vi "SET_FIRE_CUSTOM.vi"(10 "argv":string[](array[string]), 11 "args":u8) -> ()   [LabVIEW 2011]
uses:
  <vilib>/Rock Robotics/WPI/DriverStation/WPI_DriverStationStatusErrorCache.ctl
  Auto_Conf.vi
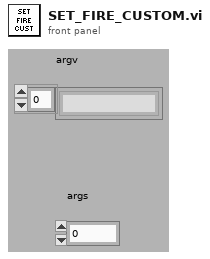
[diagram p1: front panel]
types:
  T1 = typedef "WPI_DriverStationStatusErrorCache.ctl" = enum16{"Get", "Set"}
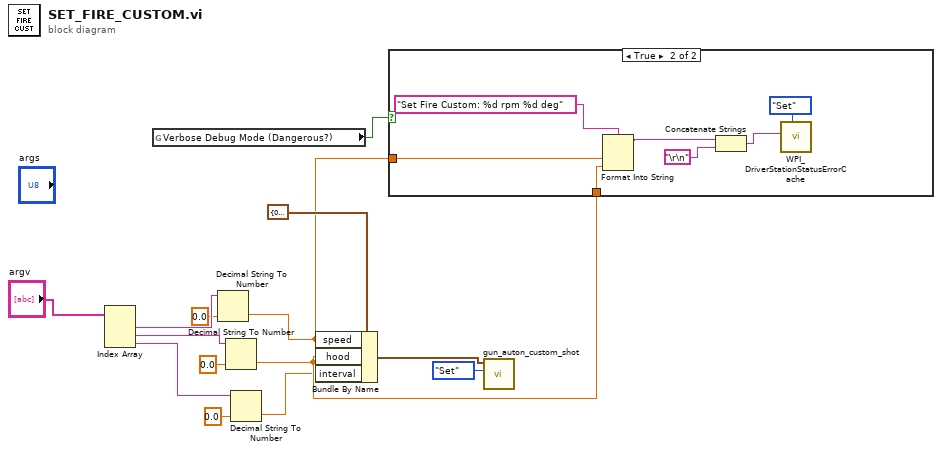
[diagram p0: block diagram]
diagram:
  n1 = Index Array(array="argv") -> (element #1=w13:string, element #2=w10:string, element #3=w2:string)  [unwired: 3 in]
  n2 = global read "Auto_Conf.vi" "Verbose Debug Mode (Dangerous?)"() -> (w6:bool)
  n3 = Decimal String To Number(string=w13, default (0L)=0.0 ("default (0 I32)")) -> (number=w5:dbl)  [unwired: 1 in, 1 out]
  n4 = Decimal String To Number(string=w10, default (0L)=0.0 ("default (0 I32)")) -> (number=w4:dbl)  [unwired: 1 in, 1 out]
  n5 = Decimal String To Number(string=w2, default (0L)=0.0 ("default (0 I32)")) -> (number=w1:dbl)  [unwired: 1 in, 1 out]
  n6 = Bundle By Name(cluster=cluster{"speed":dbl, "hood":dbl, "interval":dbl} {"speed"=0.0, "hood"=0.0, "interval"=0.0} ("shot params"), "speed"=w5, "hood"=w4, "interval"=w1) -> (w8:cluster{"speed":dbl, "hood":dbl, "interval":dbl})
  n7 = case shown="True" w6 {
    tunnel: w5 -> [_ w16]
    tunnel: w4 -> [_ w15]
    frame False {
    }
    frame True {
      n8 = Format Into String(format string="Set Fire Custom: %d rpm %d deg" ("string"), w16, w15) -> (resulting string=w18:string)  [unwired: 2 in, 1 out]
      n9 = Concatenate Strings(w18, "\r\n") -> (w20:string)
      n10 = call <vilib>:"WPI_DriverStationStatusErrorCache.vi"("StatusErrorCacheOp"=WPI_DriverStationStatusErrorCache."Set", "Error String"=w20) -> ()  [unwired: 10 out]
    }
  }
  n11 = call "gun_auton_custom_shot.vi"("data_store_mode"=enum16{"Set", "Get"}."Set", "shot params"=w8) -> ()  [unwired: 9 in, 1 out]
